vi "Init Device.vi"(8 "error in (no error)":errorcluster, 11 "Laser Quantum in":refnum<class "Laser Quantum.lvclass">) -> (0 "error out":errorcluster, 3 "Laser Quantum out":refnum<class "Laser Quantum.lvclass">)   [LabVIEW 2018, in "Laser Quantum.lvlib" / "Laser Quantum.lvclass"]
uses:
  Laser Quantum.lvclass
  Laser Quantum.lvclass/Laser Quantum.ctl
  <vilib>/Instr/_visa.llb/VISA Configure Serial Port (Instr).vi
  Resources/GLOBAL/GLOBAL Debug.vi
  <vilib>/Utility/error.llb/Error Cluster From Error Code.vi
  <vilib>/ErrorRing/Error Ring.xnode
  Device/Device.lvclass
  Laser Quantum.lvlib
panel:
  out "VISA resource name out":refnum<visa-resource-name>
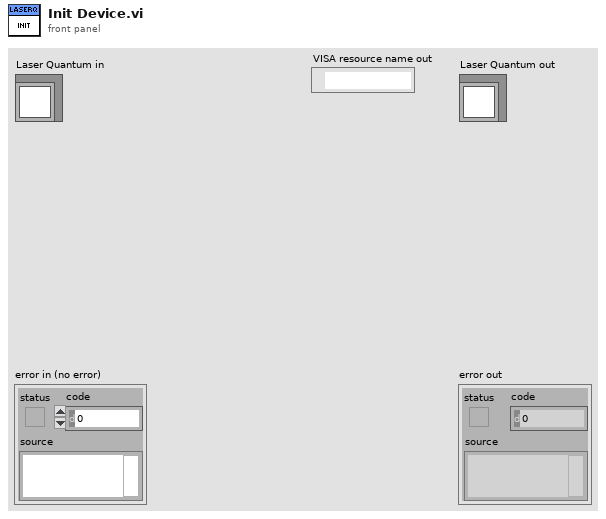
[diagram p1: front panel]
types:
  T1 = typedef "Laser Configuration.ctl" = cluster{"Serial Port":refnum<visa-resource-name>, "Laser Type":enum16{"Disable", "Laser Quantum", "Coherent OBIS", "PRM1-Z8", "Coherent HOPS"}, "Polarizer Amplitude":dbl, "Polarizer Theta Zero":dbl, "Wavelength":u16}
  T2 = enum16{"Disable", "Laser Quantum", "Coherent OBIS", "PRM1-Z8", "Coherent HOPS"}
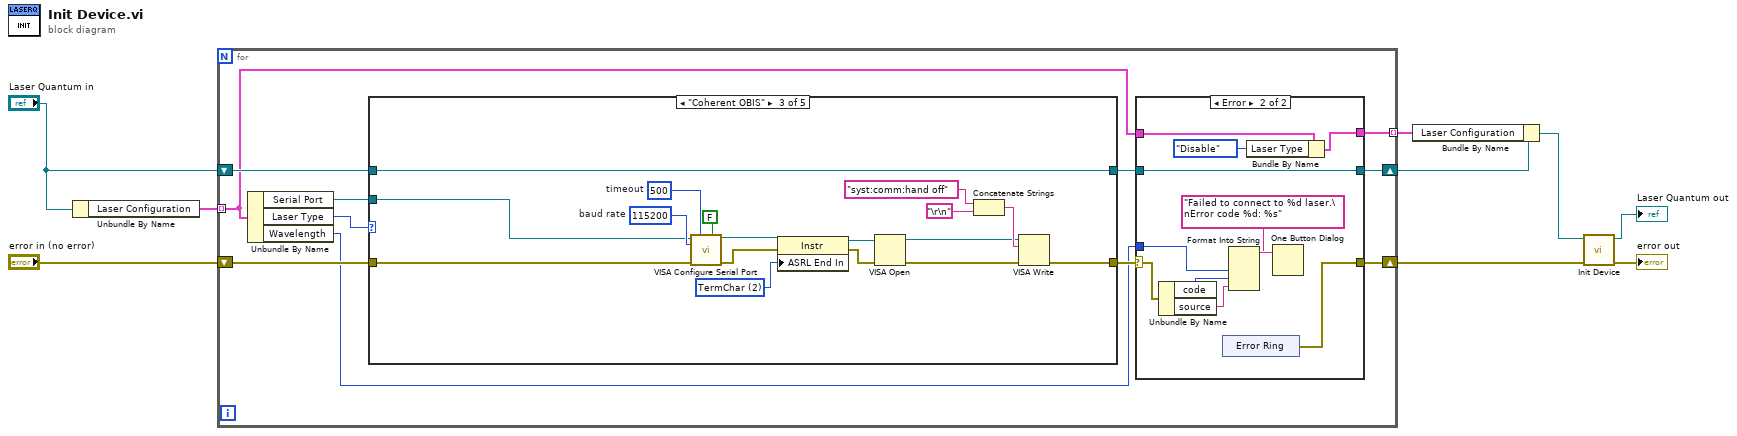
[diagram p0: block diagram]
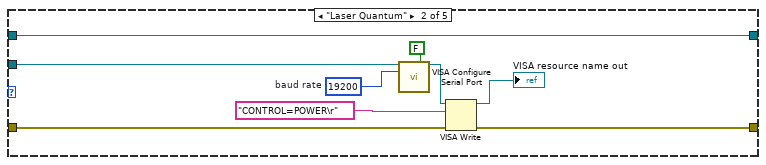
[diagram p4: hidden frame]
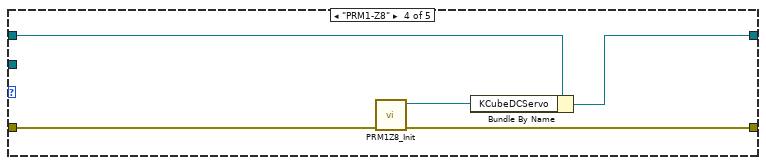
[diagram p5: hidden frame]
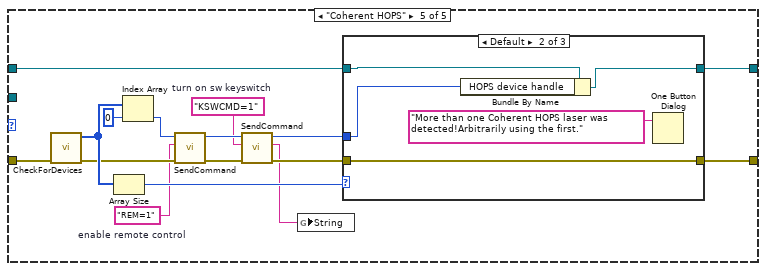
[diagram p6: hidden frame]
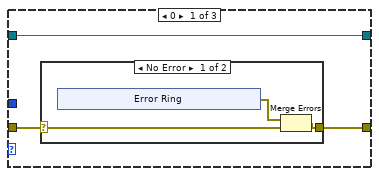
[diagram p7: hidden frame]
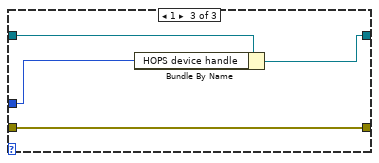
[diagram p9: hidden frame]
diagram:
  n1 = Unbundle By Name("Laser Quantum in") -> ("Laser Configuration"=w7:T1[])
  n2 = for {
    tunnel: w7 -> [w12] mode=indexing
    shift-right: [w15] -> w5
    shift-left: "error in (no error)" -> [w19]
    shift-right: [w13] -> w3
    shift-left: "Laser Quantum in" -> [w17]
    tunnel: [w11] -> w1 mode=indexing
    n3 = Unbundle By Name(w12) -> ("Serial Port"=w20:refnum<visa-resource-name>, "Laser Type"=w18:T2, "Wavelength"=w10:u16)
    n4 = case shown="\"Coherent OBIS\"" w18 {
      tunnel: w20 -> [_ w45 w50 _ _]
      tunnel: w19 -> [w37 w41 w49 w68 w84]
      tunnel: [w37 w40 w58 w67 w80] -> w16
      tunnel: w17 -> [w36 w38 w57 w66 w79]
      tunnel: [w36 w38 w57 w65 w78] -> w14
      frame "Disable", Default {
      }
      frame "Laser Quantum" {
        w43 = u32 19200  # baud rate
        n5 = call-poly "VISA Configure Serial Port"("VISA resource name"=w45, "Enable Termination\nChar (T)"=FALSE ("Enable Termination\nChar (T)"), "baud rate (9600)"=w43) -> ("VISA resource name out"=w46:refnum<visa-resource-name>)  [unwired: 11 in, 1 out]
        n6 = VISA Write(VISA resource name=w46, write buffer="CONTROL=POWER\r", error in (no error)=w41) -> (VISA resource name out=→"VISA resource name out":refnum<visa-resource-name>, error out=w40:errorcluster)  [unwired: 1 out]
      }
      frame "Coherent OBIS" {
        w51 = u16 2 items=["None", "Last Bit", "TermChar"] ("Serial Settings:End Mode for Reads")
        w56 = u32 500  # timeout
        w59 = u32 115200  # baud rate
        n7 = call-poly "VISA Configure Serial Port"("VISA resource name"=w50, "timeout (10sec)"=w56, "Enable Termination\nChar (T)"=FALSE ("Enable Termination\nChar (T)"), "baud rate (9600)"=w59, "error in (no error)"=w49) -> ("VISA resource name out"=w55:refnum<visa-resource-name>, "error out"=w52:errorcluster)  [unwired: 9 in]
        n8 = property class="Instr"(reference=w55, error in=w52, "ASRL End In"=w51) -> (reference out=w54:refnum<visa-resource-name>, error out=w53:errorcluster)
        n9 = VISA Open(error in (no error)=w53, VISA resource name=w54) -> (VISA resource name=w47:refnum<visa-resource-name>, error out=w48:errorcluster)  [unwired: 3 in]
        n10 = Concatenate Strings("syst:comm:hand off" ("write to laser"), "\r\n") -> (w63:string)
        n11 = VISA Write(VISA resource name=w47, write buffer=w63, error in (no error)=w48) -> (error out=w58:errorcluster)  [unwired: 2 out]
      }
      frame "PRM1-Z8" {
        n12 = call "PRM1Z8_Init.vi"("error in (no error)"=w68) -> ("error out"=w67:errorcluster, "reference out"=w64:refnum<k24>)  [unwired: 9 in]
        n13 = Bundle By Name(cluster=w66, "KCubeDCServo"=w64) -> (w65:refnum<class "Laser Quantum.lvclass">)
      }
      frame "Coherent HOPS" {
        w69 = "KSWCMD=1"  # turn on sw keyswitch
        w75 = "REM=1"  # enable remote control
        n14 = call "CheckForDevices.vi"("error in"=w84) -> ("error out"=w77:errorcluster, "Device Handles"=w81:u64[])  [unwired: 6 in, 1 out]
        n15 = Array Size(array=w81) -> (size(s)=w82:i32)
        n16 = Index Array(array=w81, index=0 ("Index")) -> (element=w76:u64)
        n17 = call "SendCommand.vi"("error in"=w77, "Command"=w75, "Device Handle"=w76) -> ("error out"=w74:errorcluster, "Dup Handle"=w71:u64)  [unwired: 3 in, 2 out]
        n18 = call "SendCommand.vi"("error in"=w74, "Command"=w69, "Device Handle"=w71) -> ("error out"=w73:errorcluster, "String"=w70:string, "Dup Handle"=w72:u64)  [unwired: 3 in, 1 out]
        n19 = global write "GLOBAL Debug.vi" "String"(w70) -> ()
        n20 = case shown="Default" w82 {
          tunnel: w72 -> [_ w96 w101]
          tunnel: w73 -> [w85 w99 w104]
          tunnel: [w87 w99 w104] -> w80
          tunnel: w79 -> [w86 w97 w102]
          tunnel: [w86 w98 w103] -> w78
          frame 0 {
            n21 = case shown="No Error" w85 {
              selector: w85 -> [w88 w95]
              tunnel: [w90 w95] -> w87
              frame No Error {
                n22 = xnode "Error Ring"() -> ("error out"=w89:errorcluster)
                n23 = Merge Errors(w89, w88) -> (w90:errorcluster)
              }
              frame Error {
              }
            }
          }
          frame Default {
            n24 = Bundle By Name(cluster=w97, "HOPS device handle"=w96) -> (w98:refnum<class "Laser Quantum.lvclass">)
            n25 = One Button Dialog(message="More than one Coherent HOPS laser was detected!Arbitrarily using the first.") -> ()  [unwired: 1 in, 1 out]
          }
          frame 1 {
            n26 = Bundle By Name(cluster=w102, "HOPS device handle"=w101) -> (w103:refnum<class "Laser Quantum.lvclass">)
          }
        }
      }
    }
    n27 = case shown="Error" w16 {
      selector: w16 -> [w23 w29]
      tunnel: [w23 w34] -> w15
      tunnel: w14 -> [w22 w33]
      tunnel: [w22 w33] -> w13
      tunnel: w12 -> [w21 w32]
      tunnel: [w21 w31] -> w11
      tunnel: w10 -> [_ w24]
      frame No Error {
      }
      frame Error {
        n28 = Unbundle By Name(w29) -> ("code"=w25:i32, "source"=w26:string)
        n29 = xnode "Error Ring"() -> ("error out"=w34:errorcluster)
        n30 = Format Into String(format string="Failed to connect to %d laser.\nError code %d: %s" ("message"), w24, w25, w26) -> (resulting string=w28:string)  [unwired: 2 in, 1 out]
        n31 = Bundle By Name(cluster=w32, "Laser Type"=T2."Disable") -> (w31:T1)
        n32 = One Button Dialog(message=w28) -> ()  [unwired: 1 in, 1 out]
      }
    }
  }
  n33 = Bundle By Name(cluster=w3, "Laser Configuration"=w1) -> (w2:refnum<class "Laser Quantum.lvclass">)
  n34 = call-parent "Init Device.vi"("error in (no error)"=w5, "Device in"=w2) -> ("error out"=→"error out":errorcluster, "Device out"=→"Laser Quantum out":refnum<class "Laser Quantum.lvclass">)  [unwired: 8 in]
